vi "FuncImg-Obtain funct data path.vi"(8 "error in":errorcluster) -> (0 "error out":errorcluster, 1 "Version index (-1 = latest version)":i32, 2 "file or folder exists?":bool, 3 "Functional data folder path":path, 5 "Experiment data folder path":path)   [LabVIEW 2013]
uses:
  Typedefs/Enum-Which file or folder.ctl
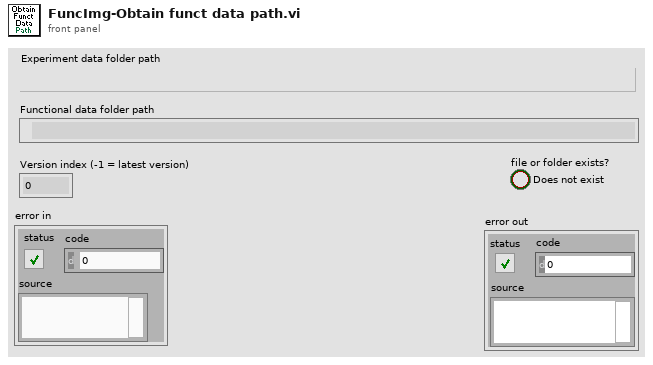
[diagram p1: front panel]
types:
  T1 = typedef "Enum-Which file or folder.ctl" = enum16{"ROI file", "Normalised ROI file", "Zplane Pockels values file", "Functional data folder"}
  T2 = typedef "Fixed strings.ctl" = cluster{"ROI file name":string, "Normalised ROI file name":string, "Zplane Pockels values file name":string, "Functional data folder name":string, "Experiment Header file name":string, "Z-stack images folder name":string, "Groups setup rel. path":string, "Groups text file rel. path":string, "TDMS files folder name (F.img)":string, "TDMS files folder name (V.acq)":string, "TDMS files folder name (Pl.acq)":string, "Cycle rel times sequence file":string, "Dynamically called VIs folder name":string, "Time Series folder base name":string}
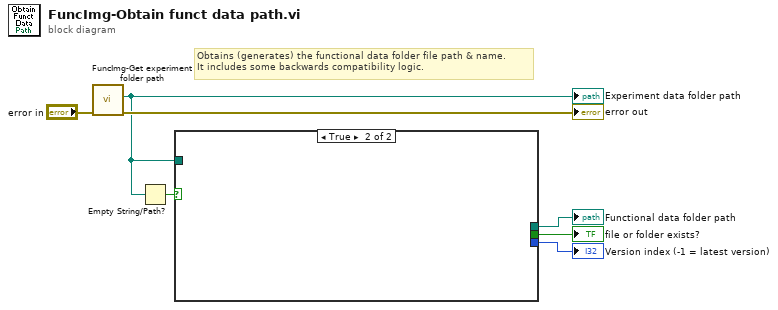
[diagram p0: block diagram]
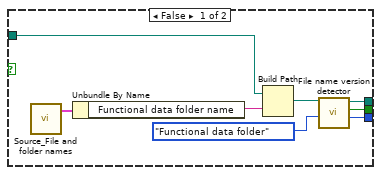
[diagram p2: hidden frame]
diagram:
  # "Obtains (generates) the functional data folder file path & name.\nIt includes some backwards compatibility logic."
  n1 = call "FuncImg-Get experiment folder path.vi"("error in (no error)"="error in") -> ("error out"=→"error out":errorcluster, "Experiment data folder path"=w1:path)  [unwired: 9 in]
  "Experiment data folder path" <- w1
  n2 = Empty String/Path?(string/path=w1) -> (empty?=w2:bool)
  n3 = case shown="True" w2 {
    tunnel: [w13 _] -> w7
    tunnel: [w11 _] -> w6
    tunnel: [w9 _] -> w5
    tunnel: w1 -> [w8 _]
    frame False {
      n4 = call "Source_File and folder names.vi"() -> ("Fixed strings"=w15:T2)  [unwired: 1 in]
      n5 = Unbundle By Name(w15) -> ("Functional data folder name"=w14:string)
      n6 = Build Path(base path=w8, name or relative path=w14) -> (appended path=w10:path)
      n7 = call "File name version detector.vi"("Which file/folder?"=Enum-Which_file_or_folder."Functional data folder", "Path in"=w10) -> ("Version index (-1 = latest version)"=w13:i32, "file or folder exists"=w9:bool, "Path out"=w11:path)  [unwired: 7 in]
    }
    frame True {
    }
  }
  "Version index (-1 = latest version)" <- w7
  "Functional data folder path" <- w6
  "file or folder exists?" <- w5
